vi "PID Main.vi"() -> ()   [LabVIEW 2019]
doc: "[Covers: REQ01]\nA aplicação deve ser desenvolvida usando a plataforma LabVIEW, já que seu aprendizado é o objetivo do projeto."
uses:
  controls/PID State.ctl
  controls/PID Data.ctl
  <vilib>/DAQmx/write.llb/DAQmx Write (Analog 1D DBL NChan 1Samp).vi
  <vilib>/DAQmx/read.llb/DAQmx Read (Analog 1D DBL NChan 1Samp).vi
  <vilib>/addons/control/pid/pid.llb/PID (DBL).vi
  <vilib>/DAQmx/miscellaneous.llb/DAQmx Fill In Error Info.vi
  <vilib>/addons/control/pid/NI_PID_pid.lvlib
panel:
  in  "Exit":bool
  in  "Stop Control":bool
  in  "Run Control":bool
  out "Status":string
  in  "Tab Control":T1(tab)
  in  "Set Point":dbl(slide)=25.0 scale=20.0..40.0
  out "Waveform Chart":T2(graph)={"Numeric <Replace Me>"=25.059130709061986, "Set Point"=25.0}
  in  "Distúrbio":dbl(slide) scale=0.0..10.0
  in  "Modo":enum16{"Real", "Simulado"}(ring)=enum."Simulado"
  in  "Update":bool
  in  "Ganhos PID":T3={"Ganho proporcional (Kc)"=5.0, "Ganho integral (Kc*Ts/Ti)"=0.008, "Ganho derivativo (Kc*Td/Ts)"=0.001}
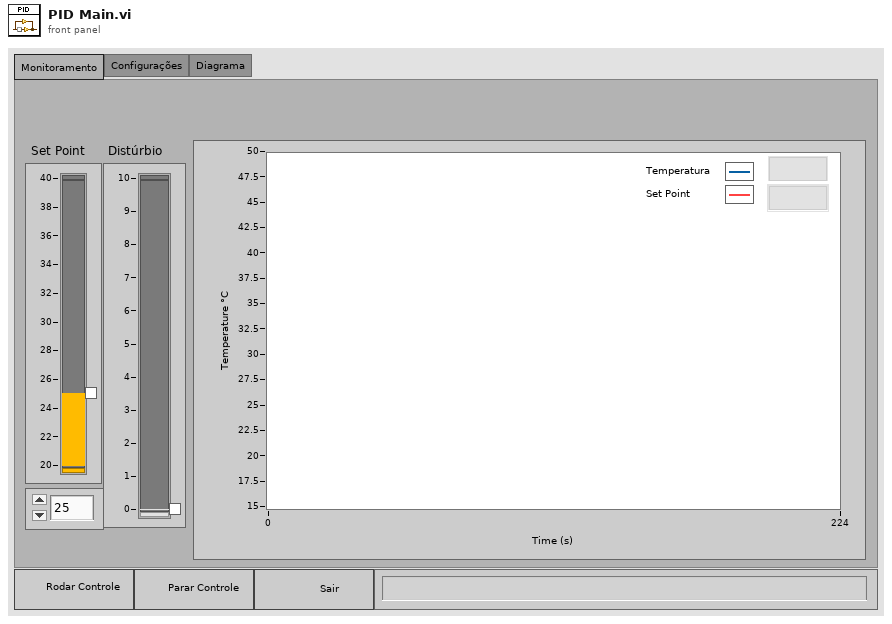
[diagram p1: front panel]
types:
  T1 = enum32{"Monitoramento", "Configurações", "Diagrama"}
  T2 = cluster{"Numeric <Replace Me>":dbl, "Set Point":dbl}
  T3 = cluster{"Ganho proporcional (Kc)":dbl, "Ganho integral (Kc*Ts/Ti)":dbl, "Ganho derivativo (Kc*Td/Ts)":dbl}
  T4 = typedef "PID Data.ctl" = cluster{"Process Variable":dbl, "Ganhos PID":cluster{"Ganho proporcional (Kc)":dbl, "Ganho integral (Kc*Ts/Ti)":dbl, "Ganho derivativo (Kc*Td/Ts)":dbl}, "Entrada Analógica":refnum<k21>, "Saída Analógica":refnum<k21>, "PWM":refnum<k21>, "Modo":enum16{"Real", "Simulado"}}
  T5 = typedef "PID State.ctl" = enum16{"Initialize", "Wait for Event", "Update PID Settings", "Start DAQ", "Control", "Stop DAQ", "Exit"}
  T6 = enum16{"Always On", "Always Off", "Off While Running"}
  T7 = cluster{"static gain":dbl, "lag (min)":dbl, "dead cycles":dbl, "load %":dbl, "deadband":dbl, "noise level %":dbl, "initial PV":dbl, "initial PV 2":dbl}
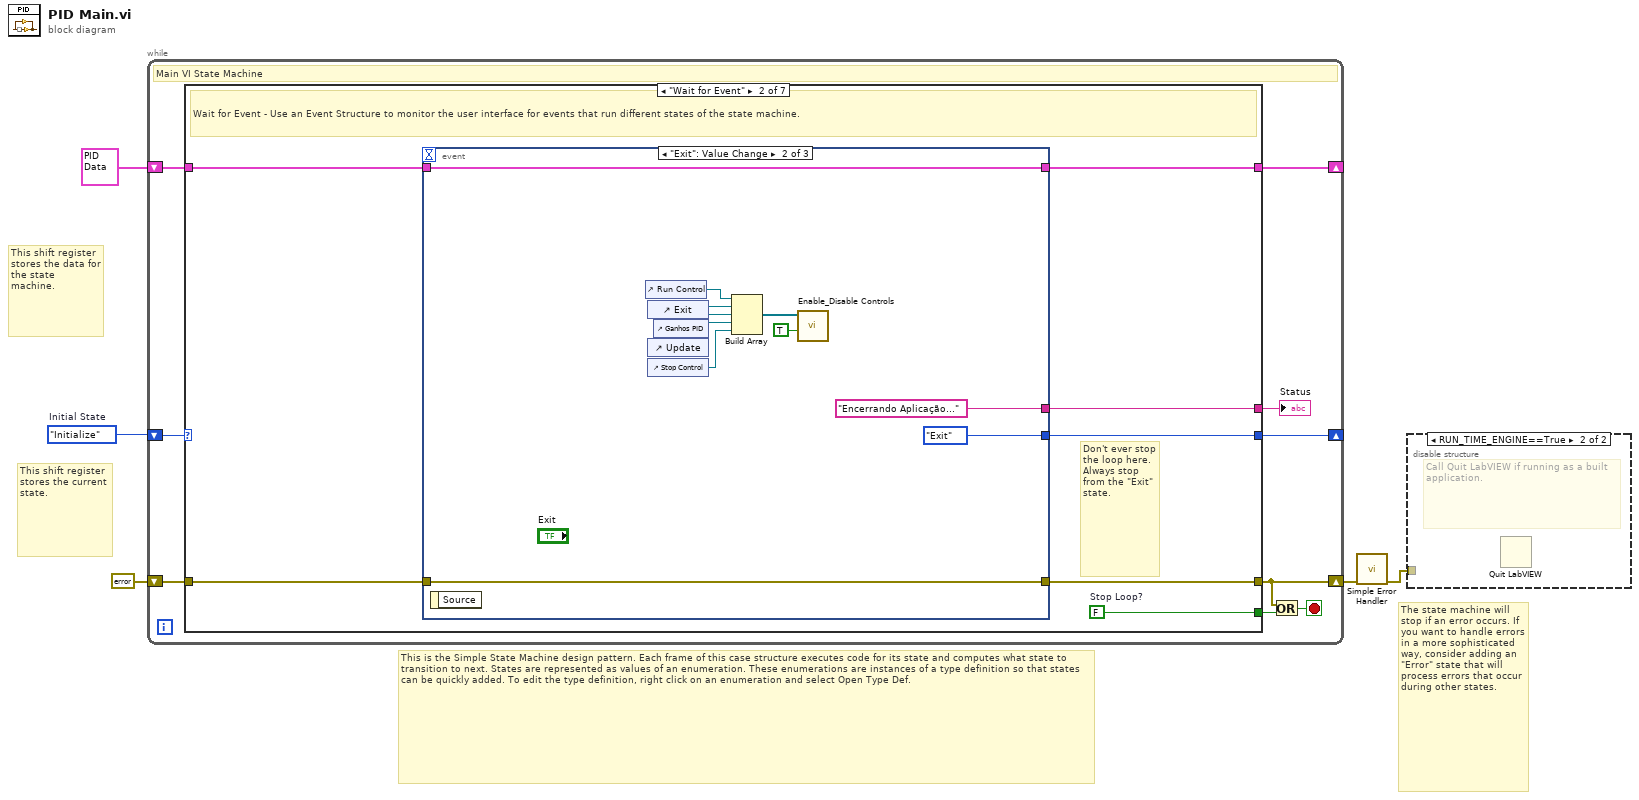
[diagram p0: block diagram]
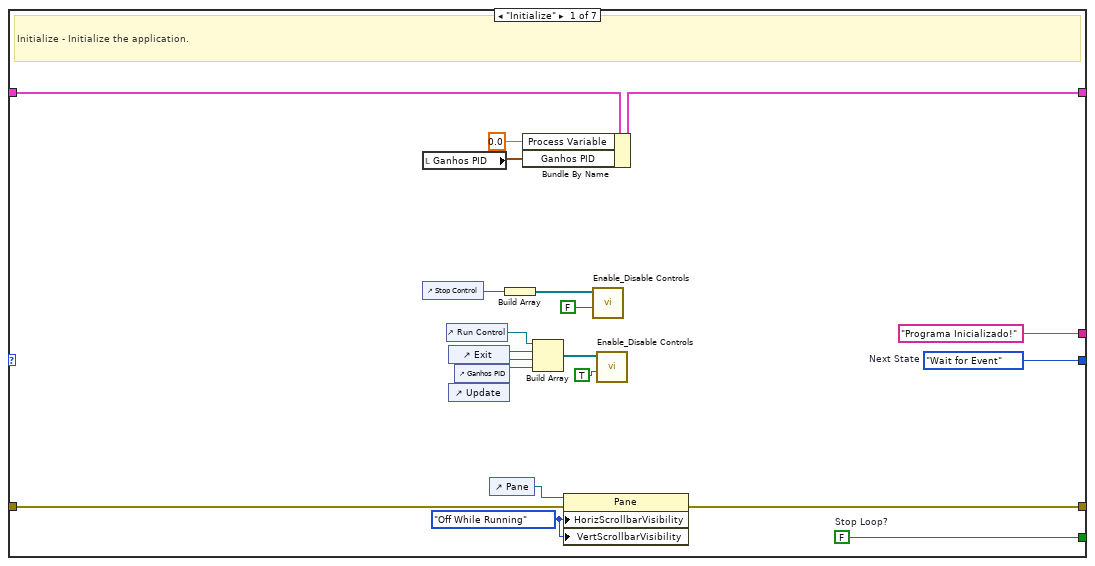
[diagram p3: hidden frame]
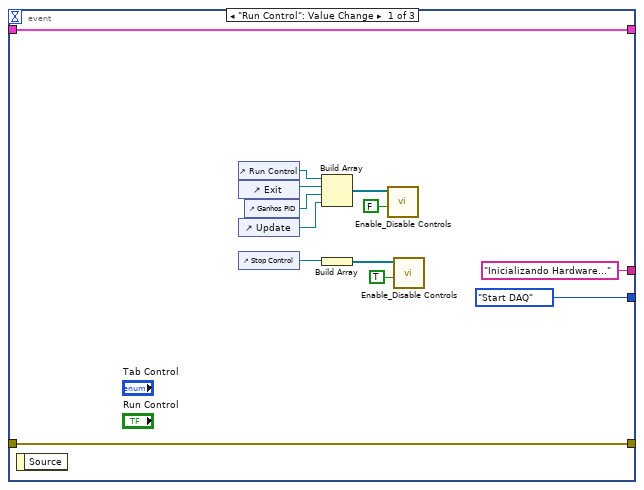
[diagram p4: hidden frame]
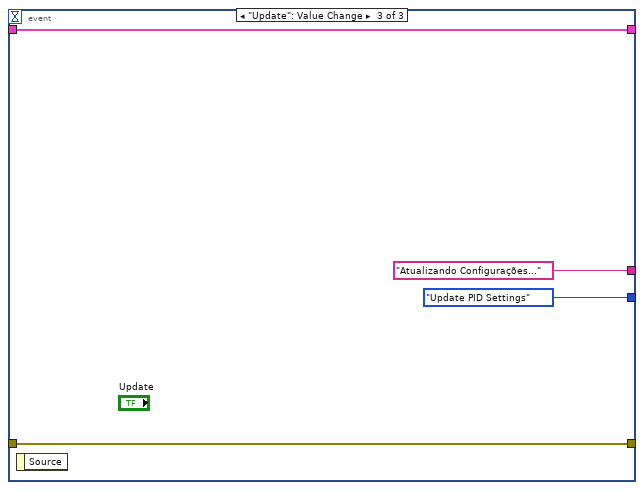
[diagram p5: hidden frame]
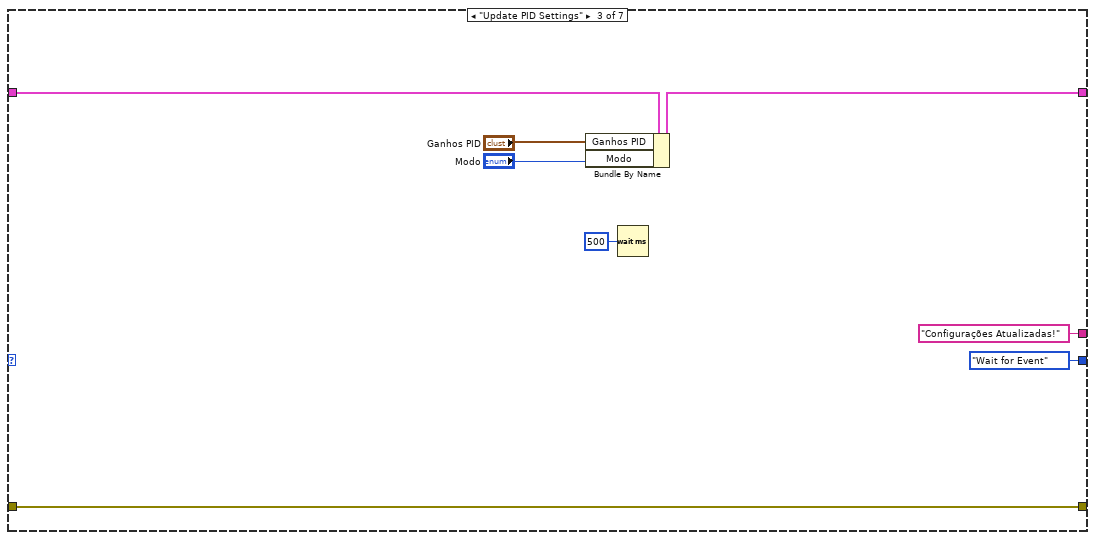
[diagram p6: hidden frame]
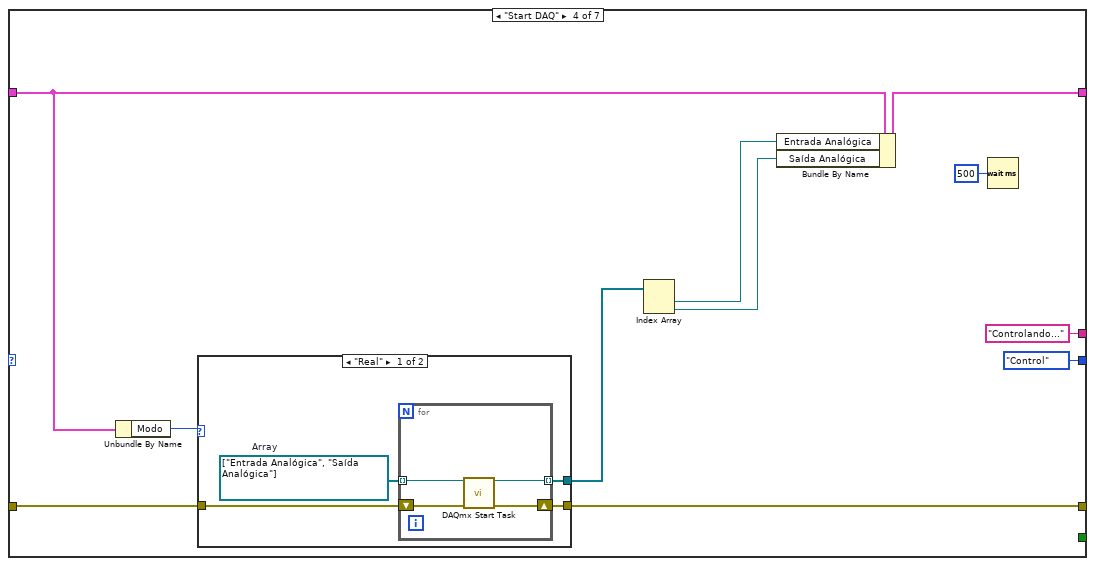
[diagram p7: hidden frame]
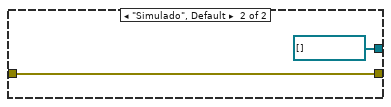
[diagram p8: hidden frame]
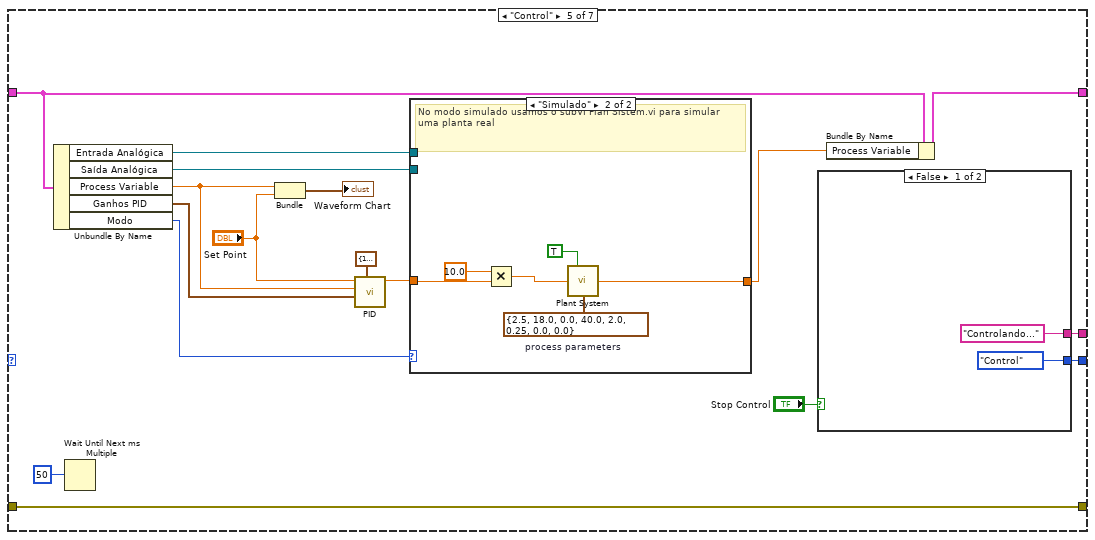
[diagram p9: hidden frame]
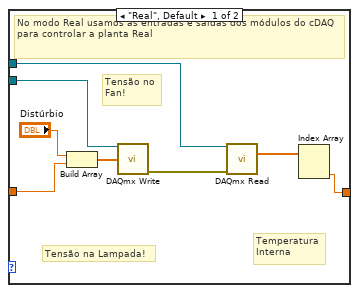
[diagram p10: hidden frame]
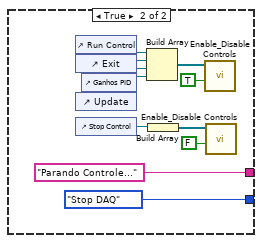
[diagram p11: hidden frame]
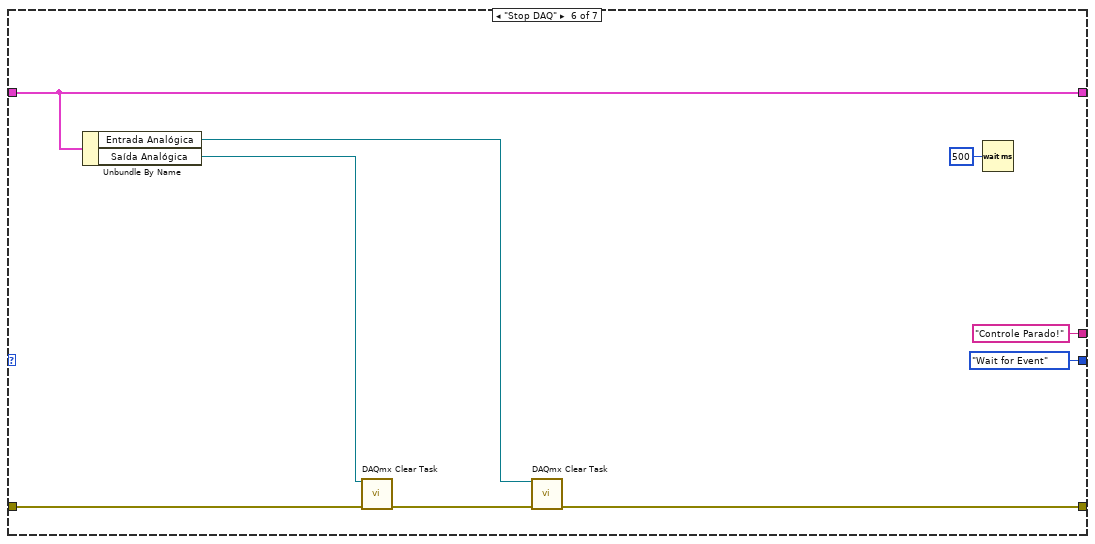
[diagram p12: hidden frame]
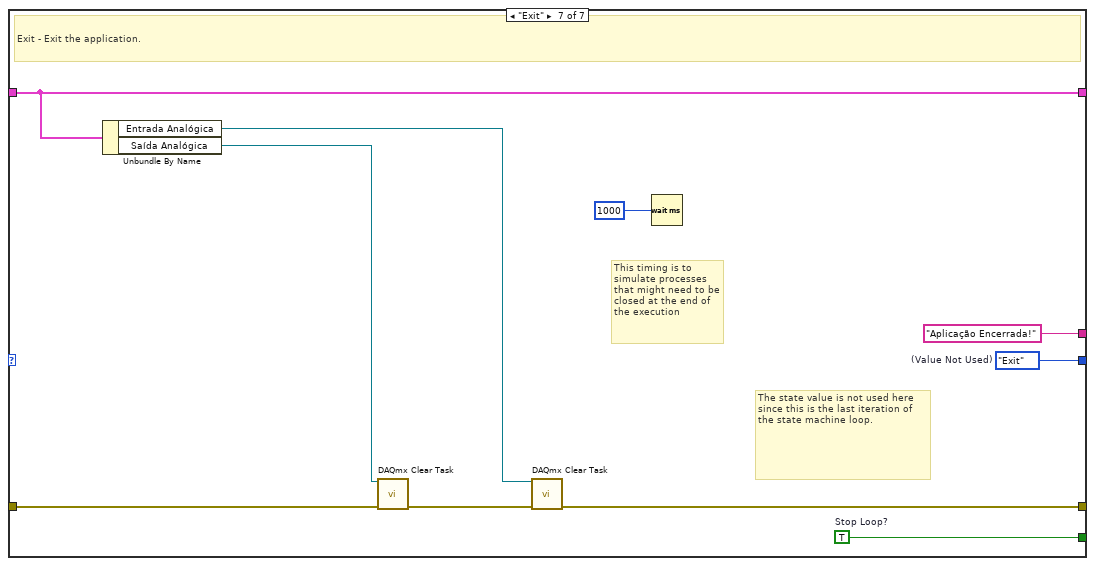
[diagram p13: hidden frame]
diagram:
  w5 = PID_State."Initialize"  # Initial State
  # "The state machine will stop if an error occurs. If you want to handle errors in a more sophisticated way, consider adding an \"Error\" state that will process errors that occur during other states."
  # "This shift register stores the data for the state machine."
  # "This is the Simple State Machine design pattern. Each frame of this case structure executes code for its state and computes what state to transition to next. States are represented as values of an enumeration. These enumerations are instances of a type definition so that states can be quickly added. To edit the type definition, right click on an enumeration and select Open Type Def."
  # "This shift register stores the current state."
  n1 = while {
    shift-right: [w13] -> _
    shift-left: w5 -> [w14]
    shift-right: [w11] -> _
    shift-left: T4 {"Process Variable"=0.0, "Ganhos PID"={"Ganho proporcional (Kc)"=0.0, "Ganho integral (Kc*Ts/Ti)"=0.0, "Ganho derivativo (Kc*Td/Ts)"=0.0}, "Entrada Analógica"="", "Saída Analógica"="", "PWM"="", "Modo"=enum."Simulado"} ("Data") -> [w12]
    shift-right: [w7] -> w2
    shift-left: errorcluster {"status"=FALSE, "code"=0, "source"=""} ("error constant") -> [w10]
    stop <- w8 stop-if-true
    # "Main VI State Machine"
    n2 = case shown="\"Wait for Event\"" w14 {
      tunnel: [w34 w41 PID_State."Wait for Event" ("(Value Not Used)") PID_State."Control" ("(Value Not Used)") w113 PID_State."Wait for Event" ("(Value Not Used)") w161] -> w13
      tunnel: [w33 w40 _ _ _ _ w160] -> w9
      tunnel: w12 -> [w32 w39 w77 w79 w108 w148 w156]
      tunnel: [w29 w38 w75 w88 w110 w148 w156] -> w11
      tunnel: w10 -> [w31 w37 w76 w84 w115 w151 w159]
      tunnel: [w24 w36 w76 w85 w115 w150 w155] -> w7
      tunnel: ["Programa Inicializado!" ("String <Replace Me>") w35 "Configurações Atualizadas!" ("String <Replace Me>") "Controlando..." ("String <Replace Me>") w114 "Controle Parado!" ("String <Replace Me>") "Aplicação Encerrada!" ("String <Replace Me>")] -> w6
      frame "Initialize" {
        w22 = T6."Off While Running" ("Horizontal Scrollbar Visibility")
        w33 = FALSE  # Stop Loop?
        w34 = PID_State."Wait for Event"  # Next State
        # "Initialize - Initialize the application."
        n3 = local read "Ganhos PID"() -> (w15:T3)
        n4 = control-ref of="Stop Control"() -> (w26:refnum<vi>)
        n5 = control-ref of="Run Control"() -> (w16:refnum<vi>)
        n6 = control-ref of="Exit"() -> (w21:refnum<vi>)
        n7 = control-ref of="Update"() -> (w19:refnum<vi>)
        n8 = control-ref of="Ganhos PID"() -> (w20:refnum<vi>)
        n9 = control-ref of="Pane"() -> (w23:refnum<vi>)
        n10 = Build Array(w26) -> (w25:refnum<vi>[])
        n11 = Bundle By Name(cluster=w32, "Process Variable"=0.0, "Ganhos PID"=w15) -> (w29:T4)
        n12 = Build Array(w16, w21, w20, w19) -> (w18:refnum<vi>[])
        n13 = property on="Property Node" class="Pane"(reference=w23, error in=w31, "HorizScrollbarVisibility"=w22, "VertScrollbarVisibility"=w22) -> (error out=w24:errorcluster)  [unwired: 1 out]
        n14 = call "Enable_Disable Controls.vi"("Enable?"=FALSE, "Array"=w25) -> ()  [unwired: 10 in]
        n15 = call "Enable_Disable Controls.vi"("Enable?"=TRUE, "Array"=w18) -> ()  [unwired: 10 in]
      }
      frame "Wait for Event" {
        w40 = FALSE  # Stop Loop?
        # "Don't ever stop the loop here. Always stop from the \"Exit\" state."
        # "Wait for Event - Use an Event Structure to monitor the user interface for events that run different states of the state machine."
        n16 = event shown="[1] \"Exit\": Value Change" {
          selector: _ -> [_ _ _]
          dyn-events: _ -> [_ _ _]
          timeout: _ -> [_ _ _]
          tunnel: [PID_State."Start DAQ" ("Next State") PID_State."Exit" ("Next State") PID_State."Update PID Settings" ("Next State")] -> w41
          tunnel: w39 -> [w54 w65 w69]
          tunnel: [w54 w65 w69] -> w38
          tunnel: w37 -> [w53 w64 w68]
          tunnel: [w53 w64 w68] -> w36
          tunnel: ["Inicializando Hardware..." "Encerrando Aplicação..." "Atualizando Configurações..."] -> w35
          event "Run Control": Value Change {
            n17 = event-data() -> ()  [unwired: 1 in, 1 out]
            n18 = control-ref of="Run Control"() -> (w44:refnum<vi>)
            n19 = control-ref of="Exit"() -> (w50:refnum<vi>)
            n20 = control-ref of="Update"() -> (w48:refnum<vi>)
            n21 = control-ref of="Stop Control"() -> (w43:refnum<vi>)
            n22 = control-ref of="Ganhos PID"() -> (w49:refnum<vi>)
            n23 = Build Array(w44, w50, w49, w48) -> (w47:refnum<vi>[])
            n24 = Build Array(w43) -> (w45:refnum<vi>[])
            n25 = call "Enable_Disable Controls.vi"("Enable?"=FALSE, "Array"=w47) -> ()  [unwired: 10 in]
            n26 = call "Enable_Disable Controls.vi"("Enable?"=TRUE, "Array"=w45) -> ()  [unwired: 10 in]
          }
          event "Exit": Value Change {
            n27 = event-data() -> ()  [unwired: 1 in, 1 out]
            n28 = control-ref of="Run Control"() -> (w55:refnum<vi>)
            n29 = control-ref of="Exit"() -> (w61:refnum<vi>)
            n30 = control-ref of="Update"() -> (w59:refnum<vi>)
            n31 = control-ref of="Stop Control"() -> (w56:refnum<vi>)
            n32 = control-ref of="Ganhos PID"() -> (w60:refnum<vi>)
            n33 = Build Array(w55, w61, w60, w59, w56) -> (w58:refnum<vi>[])
            n34 = call "Enable_Disable Controls.vi"("Enable?"=TRUE, "Array"=w58) -> ()  [unwired: 10 in]
          }
          event "Update": Value Change {
            n35 = event-data() -> ()  [unwired: 1 in, 1 out]
          }
        }
      }
      frame "Update PID Settings" {
        n36 = Bundle By Name(cluster=w77, "Ganhos PID"="Ganhos PID", "Modo"="Modo") -> (w75:T4)
        n37 = Wait (ms)(milliseconds to wait=u32 500) -> ()  [unwired: 1 out]
      }
      frame "Start DAQ" {
        n38 = Unbundle By Name(w79) -> ("Modo"=w78:enum16{"Real", "Simulado"})
        n39 = case shown="\"Real\"" w78 {
          tunnel: [w91 w98] -> w85
          tunnel: w84 -> [w90 w98]
          tunnel: [w89 refnum<k21>[] []] -> w82
          frame "Real" {
            w92 = refnum<k21>[] ["Entrada Analógica", "Saída Analógica"]  # Array
            n40 = for {
              tunnel: w92 -> [w96] mode=indexing
              tunnel: [w95] -> w89 mode=indexing
              shift-right: [w94] -> w91
              shift-left: w90 -> [w93]
              n41 = call <vilib>:"DAQmx Start Task.vi"("task/channels in"=w96, "error in"=w93) -> ("task out"=w95:refnum<k21>, "error out"=w94:errorcluster)  [unwired: 12 in]
            }
          }
          frame "Simulado", Default {
          }
        }
        n42 = Index Array(array=w82) -> (element #1=w81:refnum<k21>, element #2=w80:refnum<k21>)  [unwired: 2 in]
        n43 = Bundle By Name(cluster=w79, "Entrada Analógica"=w81, "Saída Analógica"=w80) -> (w88:T4)
        n44 = Wait (ms)(milliseconds to wait=u32 500) -> ()  [unwired: 1 out]
      }
      frame "Control" {
        n45 = Unbundle By Name(w108) -> ("Entrada Analógica"=w100:refnum<k21>, "Saída Analógica"=w102:refnum<k21>, "Process Variable"=w107:dbl, "Ganhos PID"=w103:T3, "Modo"=w99:enum16{"Real", "Simulado"})
        n46 = Wait Until Next ms Multiple(millisecond multiple=u32 50 ("unsigned 32bit integer")) -> ()  [unwired: 1 out]
        n47 = Bundle("Process Variable"=w107, "Set Point"="Set Point") -> (→"Waveform Chart":cluster{"Process Variable":dbl, "Set Point":dbl})  [unwired: 1 in]
        n48 = call-poly <vilib>:"PID.vi"("output range"=cluster{"output high":dbl, "output low":dbl} {"output high"=10.0, "output low"=-10.0}, "PID gains"=w103, "process variable"=w107, "setpoint"="Set Point") -> ("output"=w105:dbl)  [unwired: 6 in, 1 out]
        n49 = case shown="\"Simulado\"" w99 {
          tunnel: [w116 w127] -> w109
          tunnel: w105 -> [w121 w126]
          tunnel: w102 -> [w120 _]
          tunnel: w100 -> [w118 _]
          frame "Real", Default {
            # "Tensão no\nFan!"
            # "Tensão na Lampada!"
            # "Temperatura\nInterna"
            # "No modo Real usamos as entradas e saídas dos módulos do cDAQ para controlar a planta Real"
            n50 = Build Array("Distúrbio", w121) -> (w122:dbl[])
            n51 = call-poly <vilib>:"DAQmx Write.vi"("task/channels in"=w120, "data"=w122) -> ("error out"=w117:errorcluster)  [unwired: 11 in, 2 out]
            n52 = call-poly <vilib>:"DAQmx Read.vi"("task/channels in"=w118, "error in"=w117) -> ("data"=w119:dbl[])  [unwired: 11 in, 2 out]
            n53 = Index Array(array=w119) -> (element #2=w116:dbl)  [unwired: 2 in, 1 out]
          }
          frame "Simulado" {
            w128 = T7 {"static gain"=2.5, "lag (min)"=18.0, "dead cycles"=0.0, "load %"=40.0, "deadband"=2.0, "noise level %"=0.25, "initial PV"=0.0, "initial PV 2"=0.0}  # process parameters
            # "No modo simulado usamos o subVI Plan Sistem.vi para simular uma planta real"
            n54 = Multiply(x=10.0, y=w126) -> (x*y=w125:dbl)
            n55 = call "Plant System.vi"("Integrator ?"=TRUE, "Plant Input"=w125, "process parameters"=w128) -> ("Plant Output"=w127:dbl)  [unwired: 12 in]
          }
        }
        n56 = case shown="False" "Stop Control" {
          tunnel: ["Controlando..." ("String <Replace Me>") "Parando Controle..." ("String <Replace Me>")] -> w114
          tunnel: [PID_State."Control" ("Next State") PID_State."Stop DAQ" ("Next State")] -> w113
          frame False {
          }
          frame True {
            n57 = control-ref of="Run Control"() -> (w135:refnum<vi>)
            n58 = control-ref of="Exit"() -> (w140:refnum<vi>)
            n59 = control-ref of="Update"() -> (w138:refnum<vi>)
            n60 = control-ref of="Stop Control"() -> (w134:refnum<vi>)
            n61 = control-ref of="Ganhos PID"() -> (w139:refnum<vi>)
            n62 = Build Array(w135, w140, w139, w138) -> (w137:refnum<vi>[])
            n63 = Build Array(w134) -> (w136:refnum<vi>[])
            n64 = call "Enable_Disable Controls.vi"("Enable?"=TRUE, "Array"=w137) -> ()  [unwired: 10 in]
            n65 = call "Enable_Disable Controls.vi"("Enable?"=FALSE, "Array"=w136) -> ()  [unwired: 10 in]
          }
        }
        n66 = Bundle By Name(cluster=w108, "Process Variable"=w109) -> (w110:T4)
      }
      frame "Stop DAQ" {
        n67 = Unbundle By Name(w148) -> ("Entrada Analógica"=w147:refnum<k21>, "Saída Analógica"=w146:refnum<k21>)
        n68 = call <vilib>:"DAQmx Clear Task.vi"("task in"=w146, "error in"=w151) -> ("error out"=w149:errorcluster)  [unwired: 13 in]
        n69 = call <vilib>:"DAQmx Clear Task.vi"("task in"=w147, "error in"=w149) -> ("error out"=w150:errorcluster)  [unwired: 13 in]
        n70 = Wait (ms)(milliseconds to wait=u32 500) -> ()  [unwired: 1 out]
      }
      frame "Exit" {
        w160 = TRUE  # Stop Loop?
        w161 = PID_State."Exit"  # (Value Not Used)
        # "This timing is to simulate processes that might need to be closed at the end of the execution"
        # "The state value is not used here since this is the last iteration of the state machine loop."
        # "Exit - Exit the application."
        n71 = Unbundle By Name(w156) -> ("Entrada Analógica"=w152:refnum<k21>, "Saída Analógica"=w153:refnum<k21>)
        n72 = call <vilib>:"DAQmx Clear Task.vi"("task in"=w153, "error in"=w159) -> ("error out"=w154:errorcluster)  [unwired: 13 in]
        n73 = call <vilib>:"DAQmx Clear Task.vi"("task in"=w152, "error in"=w154) -> ("error out"=w155:errorcluster)  [unwired: 13 in]
        n74 = Wait (ms)(milliseconds to wait=u32 1000) -> ()  [unwired: 1 out]
      }
    }
    "Status" <- w6
    n75 = Or(x=w7, y=w9) -> (x .or. y?=w8:bool)
  }
  n76 = call <vilib>:"Simple Error Handler.vi"("error in (no error)"=w2) -> ("error out"=w1:errorcluster)  [unwired: 4 in, 4 out]
  n77 = disable-structure "Conditional Disable Structure" shown="RUN_TIME_ENGINE==True" {
    disable-tunnel: w1 -> [_ _]
    frame condition #0 (active) {
    }
    frame condition #1 {
      # "Call Quit LabVIEW if running as a built application."
      n78 = Quit LabVIEW() -> ()  [unwired: 1 in]
    }
  }
